vi "Timing - Interruptible Timer.vi"(6 "Time":refnum<vi>, 8 "error in (no error)":errorcluster, 10 "Update UI?":bool, 11 "Wait (s)":i32) -> (0 "error out":errorcluster, 2 "Time Elapsed":u32, 3 "Aborted?":bool)   [LabVIEW 2014]
uses:
  <vilib>/Platform/TimedLoop/XDataNode/timing_clust.ctl
  <vilib>/Platform/TimedLoop/XDataNode/nitl_modes.ctl
  <vilib>/Platform/TimedLoop/XDataNode/wakeup.ctl
  <vilib>/platform/TimedLoop/XDataNode/XDataNode.xnode
  <vilib>/Platform/TimedLoop/XDataNode/XDNodeRunTimeDep.lvlib
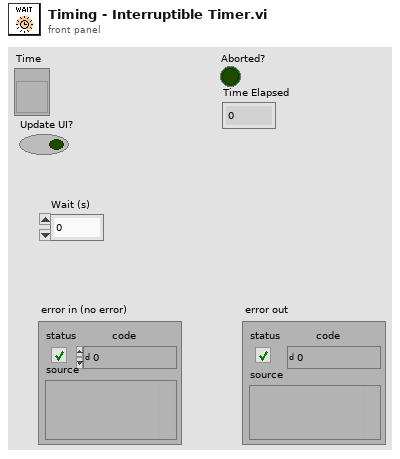
[diagram p1: front panel]
types:
  T1 = typedef "XDNodeRunTimeDep.lvlib/timing_clust.ctl" = cluster{"Expected End [f-1]":u64, "Actual End [f-1]":u64, "Finished Late? [f-1]":bool, "Expected End [i-1]":u64, "Actual End [i-1]":u64, "Finished Late? [i-1]":bool, "Expected Start [i]":u64, "Actual Start [i]":u64, "Expected Start [f]":u64, "Actual Start [f]":u64, "Source Name":string, "Structure Name":string, "Period":i64, "Deadline":i64, "Offset":i64, "Start":i64, "Priority":i32, "Timeout":i32, "Mode":T2, "Wakeup Reason":T3, "Error":errorcluster, "Source Type":string, "Secondary Source Type":string, "Global End Time":u64, "Global Start Time":u64, "Frame Duration":u64, "Iteration Duration":u64, "Assigned CPU":i32, "I/O Scan Engine Mode":u32}
  T2 = typedef "XDNodeRunTimeDep.lvlib/nitl_modes.ctl" = enum32{"No Change", "Process missed periods, maintain original phase", "Discard missed periods, maintain original phase", "Process missed periods, ignore original phase", "Discard missed periods, ignore original phase"}
  T3 = typedef "XDNodeRunTimeDep.lvlib/wakeup.ctl" = enum32{"Normal", "Aborted", "Asynchronous wakeup", "Timing source error", "Timed loop error", "Timeout"}
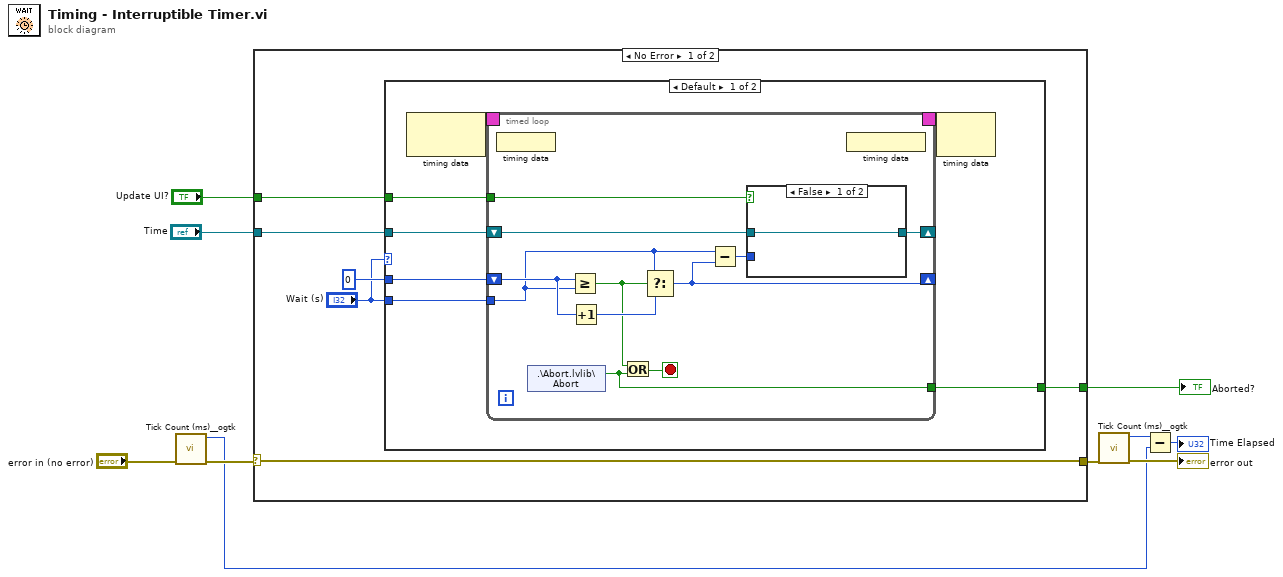
[diagram p0: block diagram]
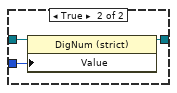
[diagram p2: hidden frame]
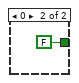
[diagram p3: hidden frame]
diagram:
  n1 = call <userlib>:"Tick Count (ms)__ogtk.vi"("error in (no error)"="error in (no error)") -> ("error out"=w8:errorcluster, "millisecond timer value"=w4:u32)  [unwired: 9 in]
  n2 = case shown="No Error" w8 {
    selector: w8 -> [w15 w44]
    tunnel: [w15 w44] -> w7
    tunnel: [w14 _] -> w10
    tunnel: "Time" -> [w13 _]
    tunnel: "Update UI?" -> [w12 _]
    frame No Error {
      n3 = case shown="Default" "Wait (s)" {
        tunnel: "Wait (s)" -> [w21 _]
        tunnel: 0 -> [w20 _]
        tunnel: [w19 FALSE ("Boolean")] -> w14
        tunnel: w13 -> [w18 _]
        tunnel: w12 -> [w17 _]
        frame Default {
          n4 = node-c288() -> (w23:T1)  [unwired: 1 in]
          n5 = timed-loop {
            tunnel: w21 -> [w28]
            shift-right: [w29] -> _
            shift-left: w20 -> [w34]
            timing: w23 -> [_]
            timing-out: [_] -> w22
            tunnel: [w30] -> w19
            shift-right: [w27] -> _
            shift-left: w18 -> [w26]
            tunnel: w17 -> [w24]
            stop <- w32 stop-if-true
            n6 = node-c288() -> ()  [unwired: 1 in]
            n7 = shared-variable ".\\Abort.lvlib\\Abort"() -> (w30:bool)  [unwired: 1 in, 1 out]
            n8 = Greater Or Equal?(x=w34, y=w28) -> (x >= y?=w31:bool)
            n9 = Increment(x=w34) -> (x+1=w33:i32)
            n10 = Or(x=w31, y=w30) -> (x .or. y?=w32:bool)
            n11 = Select(t=w28, s=w31, f=w33) -> (s? t:f=w29:i32)
            n12 = Subtract(x=w28, y=w29) -> (x-y=w25:i32)
            n13 = case shown="False" w24 {
              tunnel: [w35 w38] -> w27
              tunnel: w26 -> [w35 w37]
              tunnel: w25 -> [_ w36]
              frame False {
              }
              frame True {
                n14 = property class="DigNum (strict)"(reference=w37, "Value"=w36) -> (reference out=w38:refnum<vi>)  [unwired: 1 in, 1 out]
              }
            }
            n15 = node-c288() -> ()  [unwired: 1 out]
          }
          n16 = node-c288(w22) -> ()  [unwired: 1 out]
        }
        frame 0 {
        }
      }
    }
    frame Error {
    }
  }
  "Aborted?" <- w10
  n17 = call <userlib>:"Tick Count (ms)__ogtk.vi"("error in (no error)"=w7) -> ("error out"=→"error out":errorcluster, "millisecond timer value"=w5:u32)  [unwired: 9 in]
  n18 = Subtract(x=w5, y=w4) -> (x-y=→"Time Elapsed":u32)
